vi "Less Than.vi"(1 "comparable 2":refnum<class "Hand with Joker.lvclass">, 2 "comparable 1":refnum<class "Hand with Joker.lvclass">) -> (0 "less?":bool)   [LabVIEW 2020, in "Hand with Joker.lvclass"]
doc: "Returns whether <b>Comparable 1</b> is less than, equal to, or greater than <b>Comparable 2</b>."
uses:
  Hand with Joker.lvclass
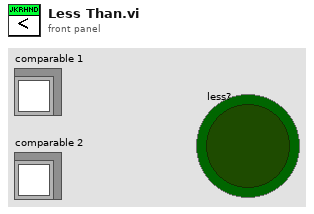
[diagram p1: front panel]
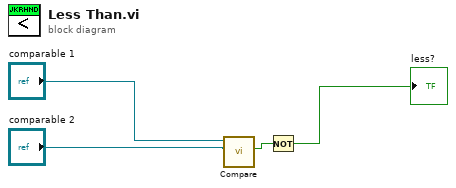
[diagram p0: block diagram]
diagram:
  n1 = call "Compare.vi"("Hand in 2"="comparable 2", "Hand in"="comparable 1") -> ("Higher?"=w2:bool)  [unwired: 7 in, 2 out]
  n2 = Not(x=w2) -> (.not. x?=→"less?":bool)
